vi "VISA_WriteRead_Anritsu.vi"(5 "waiting(ms)":u32=1, 7 "VISA_CMD":string="SYST:PRES", 8 "error in":errorcluster, 11 "VISA in":refnum<visa-resource-name>) -> (0 "error out":errorcluster, 2 "Response":string, 3 "VISA out":refnum<visa-resource-name>)   [LabVIEW 2023, in "Anritsu.lvlib"]
uses:
  Anritsu.lvlib
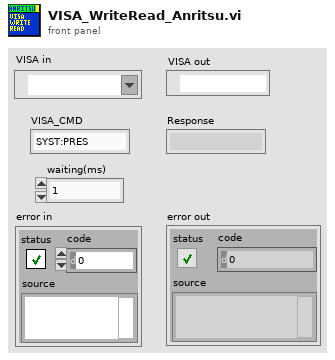
[diagram p1: front panel]
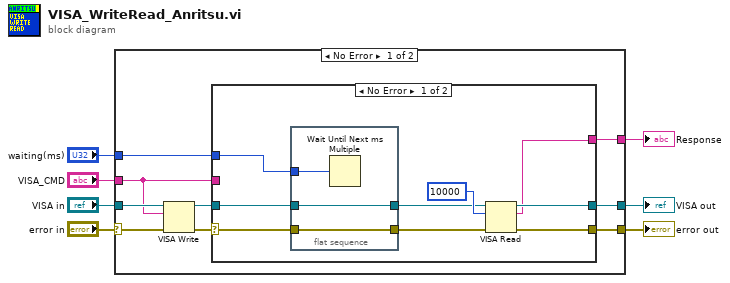
[diagram p0: block diagram]
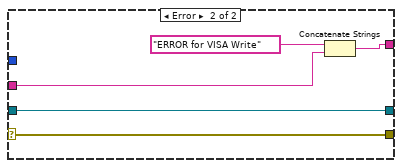
[diagram p2: hidden frame]
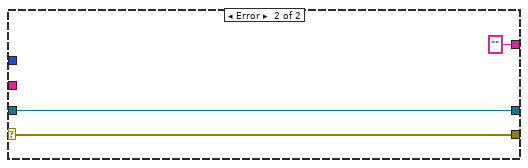
[diagram p3: hidden frame]
diagram:
  n1 = case shown="No Error" "error in" {
    selector: "error in" -> [w16 w35]
    tunnel: "VISA in" -> [w15 w36]
    tunnel: "VISA_CMD" -> [w8 _]
    tunnel: [w13 w36] -> w4
    tunnel: [w12 w35] -> w3
    tunnel: [w10 ""] -> w2
    tunnel: "waiting(ms)" -> [w9 _]
    frame No Error {
      n2 = VISA Write(VISA resource name=w15, write buffer=w8, error in (no error)=w16) -> (VISA resource name out=w14:refnum<visa-resource-name>, error out=w11:errorcluster)  [unwired: 1 out]
      n3 = case shown="No Error" w11 {
        selector: w11 -> [w21 w29]
        tunnel: w14 -> [w22 w30]
        tunnel: [w24 w30] -> w13
        tunnel: [w23 w29] -> w12
        tunnel: [w17 w31] -> w10
        tunnel: w9 -> [w18 _]
        tunnel: w8 -> [_ w32]
        frame No Error {
          n4 = flat-sequence {
            tunnel: w22 -> [w27]
            tunnel: w21 -> [w28]
            tunnel: [w28] -> w20
            tunnel: [w27] -> w19
            tunnel: w18 -> [w26]
            frame #0 {
              n5 = Wait Until Next ms Multiple(millisecond multiple=w26) -> ()  [unwired: 1 out]
            }
          }
          n6 = VISA Read(VISA resource name=w19, byte count=u32 10000 ("byte count (0)"), error in (no error)=w20) -> (VISA resource name out=w24:refnum<visa-resource-name>, read buffer=w17:string, error out=w23:errorcluster)  [unwired: 1 out]
        }
        frame Error {
          n7 = Concatenate Strings("ERROR for VISA Write", w32) -> (w31:string)
        }
      }
    }
    frame Error {
    }
  }
  "VISA out" <- w4
  "error out" <- w3
  "Response" <- w2
